vi "Stop Core.vi"(10 "final error code":i32, 11 "CS++DeviceGUIActor in":refnum<class "CS++DSCAlarmViewer.lvclass">) -> (3 "CS++DeviceGUIActor out":refnum<class "CS++DSCAlarmViewer.lvclass">)   [LabVIEW 2015, in "CS++DSCAlarmViewer.lvlib" / "CS++DSCAlarmViewer.lvclass"]
doc: "(<B>Filename</B>: Actor Framework.lvlib:Actor.lvclass:Stop Core.vi)\n\nDefines what the actor does before it stops. Use the <B>final error code</B> input to determine whether the actor shut down in response to an error.\n\nBy default, this method does nothing. A descendant class may override it to define behavior, such as shutting down any processes the actor initiated in its override of the Actor Core method."
uses:
  CS++DSCAlarmViewer.lvclass
  CSPP_Core/Actors/CS++GUIActor/CS++GUIActor.lvclass
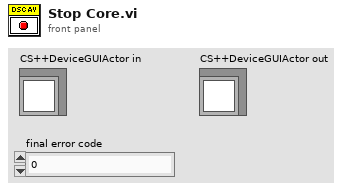
[diagram p1: front panel]
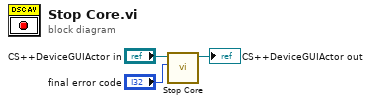
[diagram p0: block diagram]
diagram:
  n1 = call-parent "Stop Core.vi"("final error code"="final error code", "CS++GUIActor in"="CS++DeviceGUIActor in") -> ("CS++GUIActor out"=→"CS++DeviceGUIActor out":refnum<class "CS++DSCAlarmViewer.lvclass">)  [unwired: 9 in]
